vi "Yield&IntervalTime.vi"(7 "barcode":string="cc", 10 "result":bool, 11 "Cluster in":T1) -> (0 "fail":string, 1 "pass":string, 2 "Yield":string, 3 "Cluster out":T1)   [LabVIEW 2013]
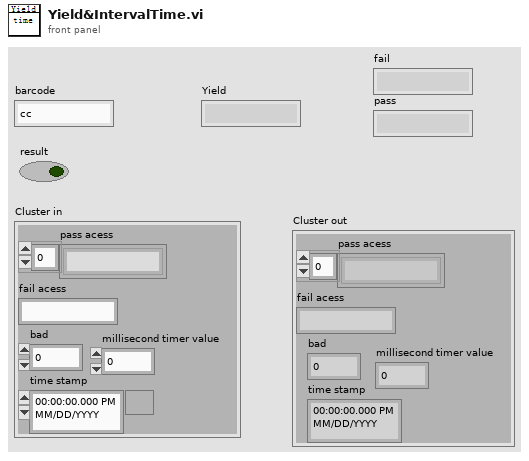
[diagram p1: front panel]
types:
  T1 = cluster{"pass acess":string[], "fail acess":string, "bad":i32, "time stamp":timestamp, "millisecond timer value":u32}
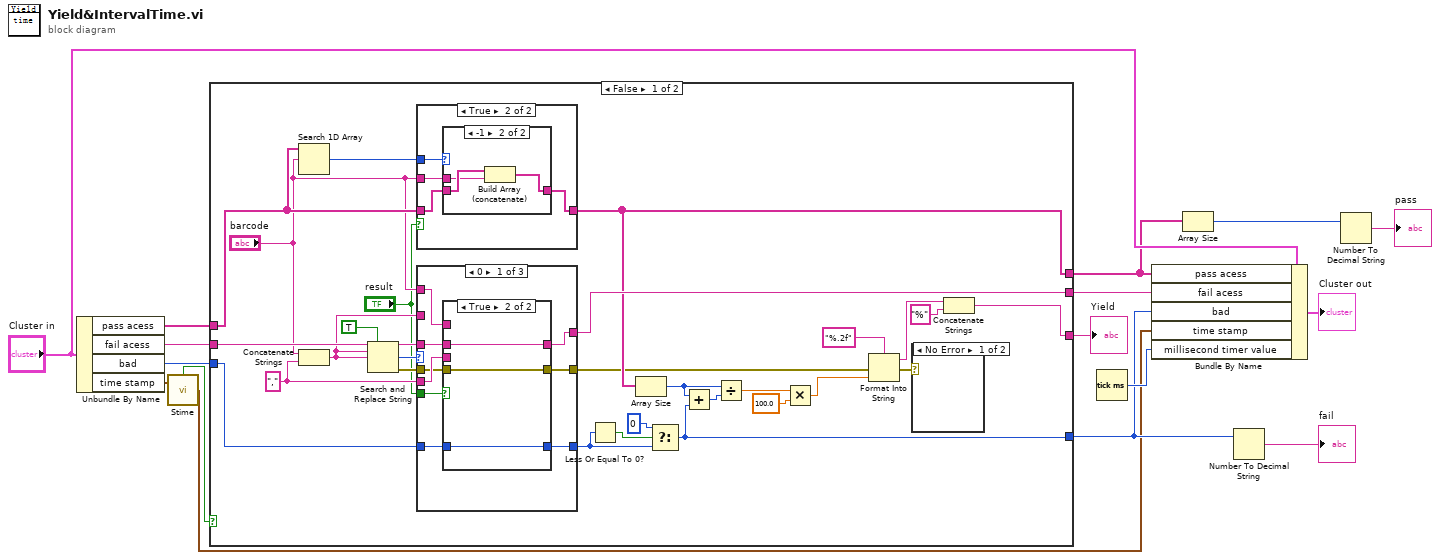
[diagram p0: block diagram]
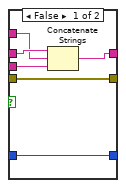
[diagram p5: hidden frame]
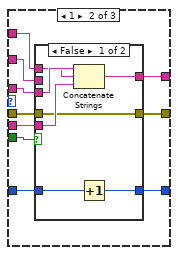
[diagram p6: hidden frame]
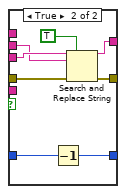
[diagram p7: hidden frame]
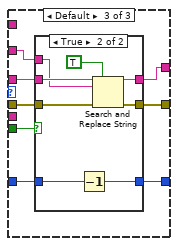
[diagram p8: hidden frame]
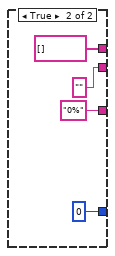
[diagram p10: hidden frame]
diagram:
  n1 = Unbundle By Name("Cluster in") -> ("pass acess"=w11:string[], "fail acess"=w12:string, "bad"=w13:i32, "time stamp"=w2:timestamp)
  n2 = call "Stime.vi"("current time"=w2) -> ("time stamp"=w3:timestamp, "x != y?"=w1:bool)  [unwired: 1 in]
  n3 = case shown="False" w1 {
    tunnel: w12 -> [w45 _]
    tunnel: [w44 "" ("result string")] -> w15
    tunnel: w11 -> [w42 _]
    tunnel: w13 -> [w41 _]
    tunnel: [w34 string[] [] ("pass acess")] -> w6
    tunnel: [w19 "0%"] -> w10
    tunnel: [w25 0 ("bad")] -> w8
    frame False {
      w35 = "," ("string")
      n4 = Search 1D Array(1D array=w42, element="barcode") -> (index of element=w43:i32)  [unwired: 1 in]
      n5 = Concatenate Strings("barcode", w35) -> (w36:string)
      n6 = Search and Replace String(replace all?=TRUE ("replace all? (F)"), input string=w45, search string=w36, replace string=w36) -> (result string=w39:string, number of replacements=w40:i32, error out=w37:errorcluster)  [unwired: 4 in, 1 out]
      n7 = case shown="True" "result" {
        tunnel: w43 -> [_ w50]
        tunnel: w42 -> [w46 w49]
        tunnel: [w46 w48] -> w34
        tunnel: "barcode" -> [_ w47]
        frame False {
        }
        frame True {
          n8 = case shown="-1" w50 {
            tunnel: w49 -> [w51 w54]
            tunnel: w47 -> [_ w52]
            tunnel: [w51 w53] -> w48
            frame Default {
            }
            frame -1 {
              n9 = Build Array (concatenate)(w54, w52) -> (w53:string[])
            }
          }
        }
      }
      n10 = case shown="0" w40 {
        tunnel: w39 -> [w63 w82 w103]
        tunnel: "barcode" -> [w62 w81 _]
        tunnel: [w61 w80 w102] -> w44
        tunnel: w41 -> [w58 w77 w105]
        tunnel: [w57 w76 w104] -> w27
        tunnel: "result" -> [w60 w79 w99]
        tunnel: w37 -> [w56 w74 w101]
        tunnel: w36 -> [_ w75 w100]
        tunnel: w35 -> [w59 w78 _]
        tunnel: [w55 w73 w98] -> w17
        frame 0 {
          n11 = case shown="True" w60 {
            tunnel: w63 -> [w69 w72]
            tunnel: w62 -> [w67 _]
            tunnel: [w68 w72] -> w61
            tunnel: w59 -> [w66 _]
            tunnel: w58 -> [w65 w71]
            tunnel: [w65 w71] -> w57
            tunnel: w56 -> [w64 w70]
            tunnel: [w64 w70] -> w55
            frame False {
              n12 = Concatenate Strings(w69, w67, w66) -> (w68:string)
            }
            frame True {
            }
          }
        }
        frame 1 {
          n13 = case shown="False" w79 {
            tunnel: w82 -> [w89 w95]
            tunnel: w81 -> [w88 _]
            tunnel: [w87 w94] -> w80
            tunnel: w78 -> [w86 _]
            tunnel: w77 -> [w85 w91]
            tunnel: [w84 w97] -> w76
            tunnel: w75 -> [_ w92]
            tunnel: w74 -> [w83 w93]
            tunnel: [w83 w90] -> w73
            frame False {
              n14 = Concatenate Strings(w89, w88, w86) -> (w87:string)
              n15 = Increment(x=w85) -> (x+1=w84:i32)
            }
            frame True {
              n16 = Decrement(x=w91) -> (x-1=w97:i32)
              n17 = Search and Replace String(replace all?=TRUE ("replace all? (F)"), input string=w95, search string=w92, error in=w93) -> (result string=w94:string, error out=w90:errorcluster)  [unwired: 4 in, 2 out]
            }
          }
        }
        frame Default {
          n18 = case shown="True" w99 {
            tunnel: w105 -> [w107 w116]
            tunnel: [w107 w115] -> w104
            tunnel: w103 -> [w108 w114]
            tunnel: [w108 w113] -> w102
            tunnel: w101 -> [w106 w112]
            tunnel: w100 -> [_ w111]
            tunnel: [w106 w109] -> w98
            frame False {
            }
            frame True {
              n19 = Decrement(x=w116) -> (x-1=w115:i32)
              n20 = Search and Replace String(replace all?=TRUE ("replace all? (F)"), input string=w114, search string=w111, error in=w112) -> (result string=w113:string, error out=w109:errorcluster)  [unwired: 4 in, 2 out]
            }
          }
        }
      }
      n21 = Less Or Equal To 0?(x=w27) -> (x <= 0?=w29:bool)
      n22 = Array Size(array=w34) -> (size(s)=w24:i32)
      n23 = Select(t=0 ("f"), s=w29, f=w27) -> (s? t:f=w25:i32)
      n24 = Add(x=w24, y=w25) -> (x+y=w23:i32)
      n25 = Divide(x=w24, y=w23) -> (x/y=w22:dbl)
      n26 = Multiply(x=w22, y=100.0) -> (x*y=w32:dbl)
      n27 = Format Into String(format string="%.2f", error in=w17, w32) -> (resulting string=w21:string, error out=w18:errorcluster)  [unwired: 1 in]
      n28 = case shown="No Error" w18 {
        frame No Error {
        }
        frame Error {
        }
      }
      n29 = Concatenate Strings(w21, "%" ("string")) -> (w19:string)
    }
    frame True {
    }
  }
  "Yield" <- w10
  n30 = Tick Count (ms)() -> (millisecond timer value=w9:u32)
  n31 = Bundle By Name(cluster="Cluster in", "pass acess"=w6, "fail acess"=w15, "bad"=w8, "time stamp"=w3, "millisecond timer value"=w9) -> (→"Cluster out":T1)
  n32 = Array Size(array=w6) -> (size(s)=w5:i32)
  n33 = Number To Decimal String(number=w8) -> (decimal integer string=→"fail":string)  [unwired: 1 in]
  n34 = Number To Decimal String(number=w5) -> (decimal integer string=→"pass":string)  [unwired: 1 in]
